vi "Logging Message Loop.vi"(8 "error in (no error)":errorcluster, 11 "Message Queues":T1) -> (0 "error out":errorcluster)   [LabVIEW 2021, in "Logging.lvlib"]
uses:
  Logging.lvlib
  Logging Configuration.ctl
  Logging State Cluster.ctl
  <vilib>/ErrorRing/Error Ring.xnode
  <vilib>/Utility/error.llb/Error Cluster From Error Code.vi
  Log State Enum.ctl
  Feed Module/Controls/Feed Module Shared Variable Cluster.ctl
  Feed Module/Feed Module.lvlib
  Settings Cluster.ctl
  Log Data Cluster.ctl
  support/Message Queue/Message Cluster.ctl
  support/Message Queue/All Message Queues.ctl
  support/Message Queue/Message Queue.lvlib
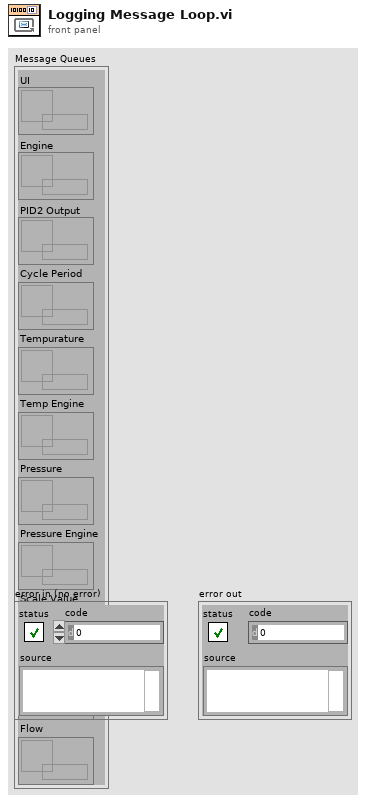
[diagram p1: front panel]
types:
  T1 = typedef "Message Queue.lvlib/All Message Queues.ctl" = cluster{"UI":refnum<queue>, "Engine":refnum<queue>, "PID2 Output":refnum<queue>, "Cycle Period":refnum<queue>, "Tempurature":refnum<queue>, "Temp Engine":refnum<queue>, "Pressure":refnum<queue>, "Pressure Engine":refnum<queue>, "Scale Value":refnum<queue>, "Pump Status":refnum<queue>, "Flow":refnum<queue>}
  T2 = typedef "Logging.lvlib/Logging State Cluster.ctl" = cluster{"State":T3, "File refnum":refnum<file>, "Start Time":timestamp, "Settings":T4, "Process Name":string, "First Record":bool}
  T3 = typedef "Logging.lvlib/Log State Enum.ctl" = enum16{"Logging", "Idle"}
  T4 = typedef "Logging.lvlib/Settings Cluster.ctl" = cluster{"Logging Configuration":T5, "Shared Variables":T6}
  T5 = typedef "Logging.lvlib/Logging Configuration.ctl" = cluster{"Log File Base Path":path}
  T6 = typedef "Feed Module.lvlib/Feed Module Shared Variable Cluster.ctl" = cluster{"PID 1 Process Variable":string, "PID 1 Output":string, "PID 1 Setpoint":string, "PID 1 Setpoint SV refnum":refnum<k21>, "PID 1 Process Variable SV refnum":refnum<k21>, "PID 1 Output SV refnum":refnum<k21>}
  T7 = enum16{"open", "replace", "create", "open or create", "replace or create", "replace or create with confirmation"}
  T8 = typedef "Logging.lvlib/Log Data Cluster.ctl" = cluster{"Time Stamp":timestamp, "PID 2 Output":dbl, "PID 2 Process Variable":dbl, "PID 1 Output":dbl}
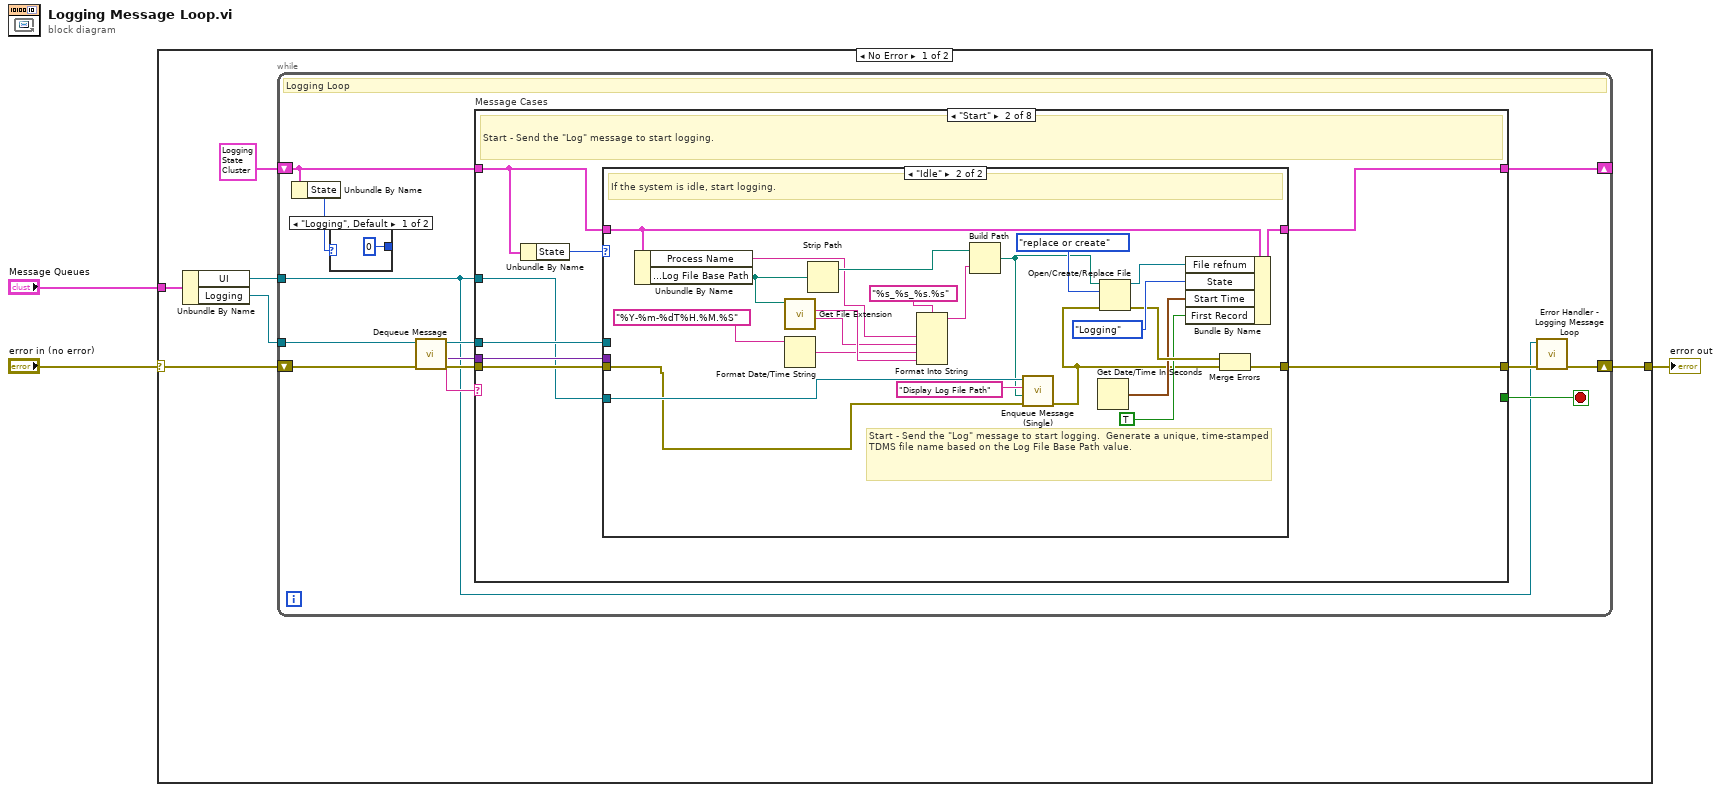
[diagram p0: block diagram]
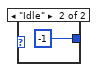
[diagram p2: hidden frame]
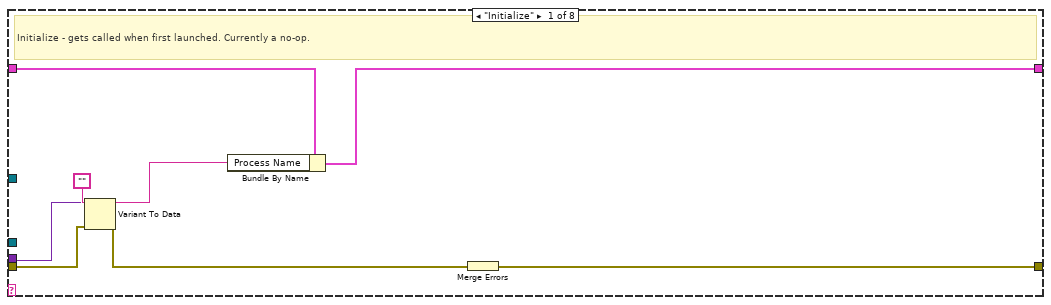
[diagram p3: hidden frame]
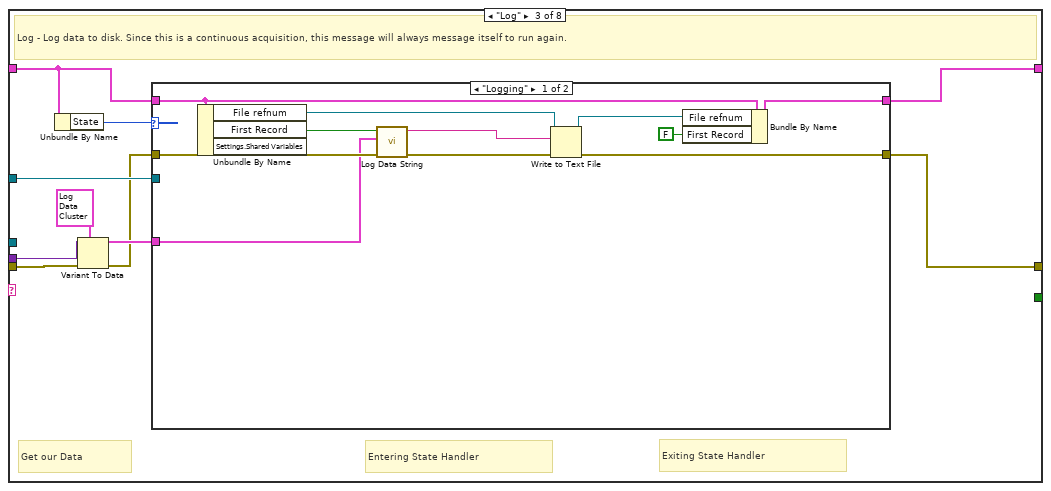
[diagram p5: hidden frame]
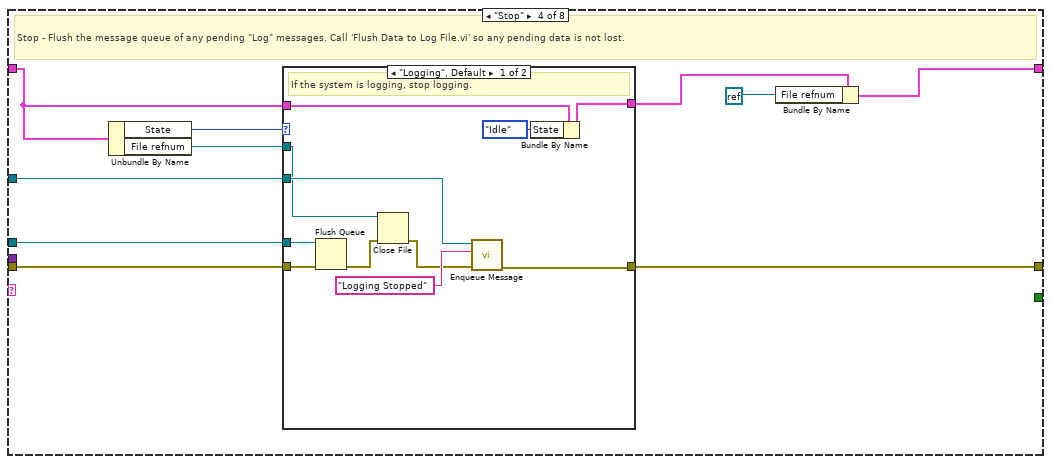
[diagram p7: hidden frame]
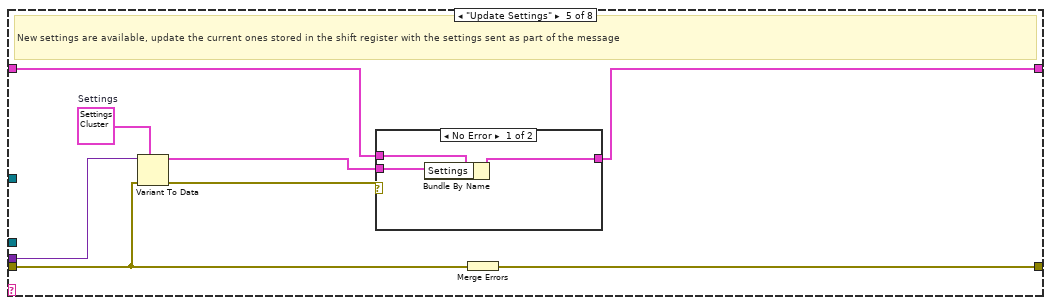
[diagram p9: hidden frame]
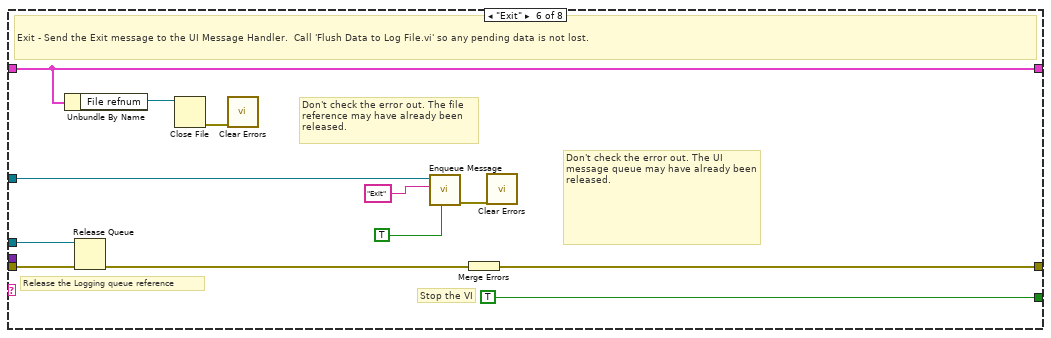
[diagram p11: hidden frame]
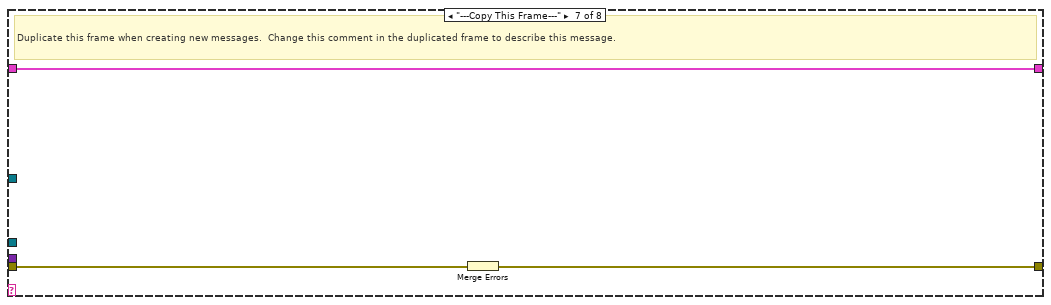
[diagram p12: hidden frame]
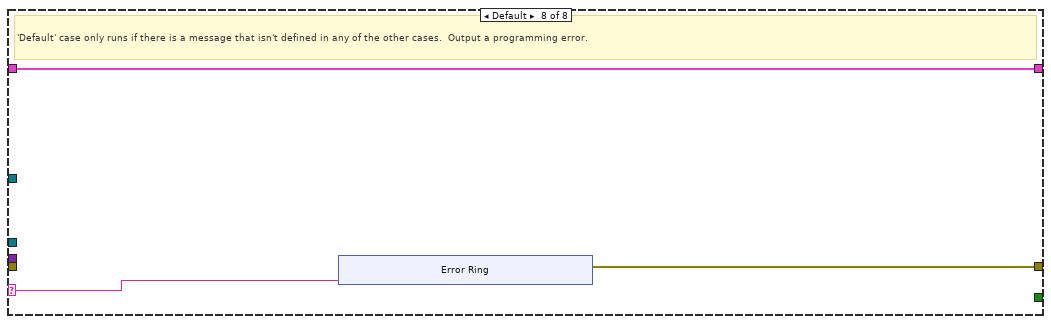
[diagram p13: hidden frame]
diagram:
  n1 = case shown="No Error" "error in (no error)" {
    selector: "error in (no error)" -> [w6 w149]
    tunnel: "Message Queues" -> [w9 _]
    tunnel: [w7 w149] -> w2
    frame No Error {
      n2 = Unbundle By Name(w9) -> ("UI"=w5:refnum<queue>, "Logging"=w8:refnum<queue>)
      n3 = while {
        tunnel: w8 -> [w16]
        shift-right: [w10] -> _
        shift-left: T2 {"State"=enum."Idle", "File refnum"=refnum, "Start Time"=timestamp(0 s since 1904-01-01), "Settings"={"Logging Configuration"={"Log File Base Path"=path ""}, "Shared Variables"={"PID 1 Process Variable"="PID1-Mettler Toledo Scale 1", "PID 1 Output"="PID1-Mettler Toledo Scale 1", "PID 1 Setpoint"="PID1-Setpoint", "PID 1 Setpoint SV refnum"="", "PID 1 Process Variable SV refnum"="", "PID 1 Output SV refnum"=""}}, "Process Name"="", "First Record"=FALSE} -> [w12]
        shift-right: [w14] -> w7
        shift-left: w6 -> [w21]
        tunnel: w5 -> [w13]
        stop <- w22 stop-if-true
        # "Logging Loop"
        n4 = Unbundle By Name(w12) -> ("State"=w11:T3)
        n5 = case shown="\"Logging\", Default" w11 {
          tunnel: [0 ("timeout in ms (-1)") -1 ("timeout in ms (-1)")] -> _
          frame "Logging", Default {
          }
          frame "Idle" {
          }
        }
        n6 = call "Dequeue Message.vi"("error in (no error)"=w21, "Message Queue"=w16) -> ("error out"=w20:errorcluster, "Message Data"=w18:variant, "Message"=w19:string, "dup Message Queue"=w17:refnum<queue>)  [unwired: 6 in]
        n7 = case "Message Cases" shown="\"Start\"" w19 {
          selector: w19 -> [_ _ _ _ _ _ _ w139]
          tunnel: w17 -> [_ w39 _ w96 _ w129 _ _]
          tunnel: w20 -> [w26 w38 w66 w97 w117 w132 w138 _]
          tunnel: [w32 w40 w73 w98 w119 w134 w136 w140] -> w15
          tunnel: w12 -> [w30 w34 w71 w91 w115 w127 w137 w141]
          tunnel: [w31 w37 w72 w95 w113 w127 w137 w141] -> w10
          tunnel: [_ _ _ _ _ TRUE _ _] -> w22
          tunnel: w18 -> [w28 w35 w70 _ w118 _ _ _]
          tunnel: w13 -> [_ w33 w74 w94 _ w133 _ _]
          frame "Initialize" {
            # "Initialize - gets called when first launched. Currently a no-op."
            n8 = Variant To Data(error in=w26, type="", Variant=w28) -> (data=w25:string, error out=w27:errorcluster)
            n9 = Bundle By Name(cluster=w30, "Process Name"=w25) -> (w31:T2)
            n10 = Merge Errors(w27) -> (w32:errorcluster)
          }
          frame "Start" {
            # "Start - Send the \"Log\" message to start logging."
            n11 = Unbundle By Name(w34) -> ("State"=w36:T3)
            n12 = case shown="\"Idle\"" w36 {
              tunnel: [w41 w65] -> w40
              tunnel: w39 -> [_ _]
              tunnel: w38 -> [w41 w43]
              tunnel: w34 -> [w42 w60]
              tunnel: [w42 w59] -> w37
              tunnel: w35 -> [_ _]
              tunnel: w33 -> [_ w47]
              frame "Logging", Default {
                # "The system is already running. Ignore the \"Start\" message."
              }
              frame "Idle" {
                # "Start - Send the \"Log\" message to start logging.  Generate a unique, time-stamped TDMS file name based on the Log File Base Path value."
                # "If the system is idle, start logging."
                n13 = Unbundle By Name(w60) -> ("Process Name"=w49:string, "Settings.Logging Configuration.Log File Base Path"=w54:path)
                n14 = call <vilib>:"Get File Extension.vi"("file"=w54) -> ("filename without extension"=w50:string, "lowercase file extension"=w62:string)  [unwired: 6 in, 3 out]
                n15 = Format Date/Time String(time format string (%c)="%Y-%m-%dT%H.%M.%S") -> (date/time string=w51:string)  [unwired: 2 in]
                n16 = Strip Path(path=w54) -> (stripped path=w53:path)  [unwired: 1 out]
                n17 = Format Into String(format string="%s_%s_%s.%s", w49, w50, w51, w62) -> (resulting string=w61:string)  [unwired: 2 in, 1 out]
                n18 = Build Path(base path=w53, name or relative path=w61) -> (appended path=w45:path)
                n19 = call "Enqueue Message (Single).vi"("error in (no error)"=w43, "Message Data"=w45, "Message"="Display Log File Path", "Message Queue"=w47) -> ("error out"=w44:errorcluster)  [unwired: 6 in, 1 out]
                n20 = Get Date/Time In Seconds() -> (seconds since 1Jan1904=w52:timestamp)
                n21 = Open/Create/Replace File(file path (use dialog)=w45, error in=w44, operation (0:open)=T7."replace or create") -> (refnum out=w56:refnum<file>, error out=w57:errorcluster)  [unwired: 3 in, 1 out]
                n22 = Bundle By Name(cluster=w60, "File refnum"=w56, "State"=Log_State_Enum."Logging", "Start Time"=w52, "First Record"=TRUE) -> (w59:T2)
                n23 = Merge Errors(w57, w44) -> (w65:errorcluster)
              }
            }
          }
          frame "Log" {
            # "Exiting State Handler"
            # "Entering State Handler"
            # "Get our Data"
            # "Log - Log data to disk. Since this is a continuous acquisition, this message will always message itself to run again."
            n24 = Unbundle By Name(w71) -> ("State"=w75:T3)
            n25 = Variant To Data(error in=w66, type=T8 {"Time Stamp"=timestamp(0 s since 1904-01-01), "PID 2 Output"=0.0, "PID 2 Process Variable"=0.0, "PID 1 Output"=0.0} ("Log Data Cluster"), Variant=w70) -> (data=w68:T8, error out=w67:errorcluster)
            n26 = case shown="\"Logging\"" w75 {
              tunnel: w67 -> [w80 w88]
              tunnel: w71 -> [w84 w87]
              tunnel: w74 -> [_ _]
              tunnel: [w86 w88] -> w73
              tunnel: [w82 w87] -> w72
              tunnel: w68 -> [w78 _]
              frame "Logging" {
                n27 = Unbundle By Name(w84) -> ("File refnum"=w85:refnum<file>, "First Record"=w76:bool)  [unwired: 1 out]
                n28 = call "Log Data String.vi"("error in (no error)"=w80, "Log Data Cluster"=w78, "First Record"=w76) -> ("error out"=w81:errorcluster, "Log Data String"=w79:string)  [unwired: 7 in]
                n29 = Write to Text File(file (use dialog)=w85, text=w79, error in=w81) -> (refnum out=w83:refnum<file>, error out=w86:errorcluster)  [unwired: 1 in, 1 out]
                n30 = Bundle By Name(cluster=w84, "File refnum"=w83, "First Record"=FALSE) -> (w82:T2)
              }
              frame "Idle", Default {
              }
            }
          }
          frame "Stop" {
            # "Stop - Flush the message queue of any pending \"Log\" messages. Call 'Flush Data to Log File.vi' so any pending data is not lost."
            n31 = Unbundle By Name(w91) -> ("State"=w93:T3, "File refnum"=w90:refnum<file>)
            n32 = case shown="\"Logging\", Default" w93 {
              tunnel: [w102 w111] -> w98
              tunnel: w97 -> [w109 w111]
              tunnel: w96 -> [w108 _]
              tunnel: w94 -> [w107 _]
              tunnel: w91 -> [w105 w110]
              tunnel: [w104 w110] -> w92
              tunnel: w90 -> [w101 _]
              frame "Logging", Default {
                # "If the system is logging, stop logging."
                n33 = Flush Queue(queue=w108, error in (no error)=w109) -> (error out=w100:errorcluster)  [unwired: 2 out]
                n34 = Close File(refnum=w101, error in=w100) -> (error out=w99:errorcluster)  [unwired: 1 out]
                n35 = call-poly "Enqueue Message.vi"("error in (no error)"=w99, "Message"="Logging Stopped", "Message Queue"=w107) -> ("error out"=w102:errorcluster)  [unwired: 7 in, 1 out]
                n36 = Bundle By Name(cluster=w105, "State"=Log_State_Enum."Idle") -> (w104:T2)
              }
              frame "Idle" {
                # "The system is already idle. Ignore the \"Stop\" message."
              }
            }
            n37 = Bundle By Name(cluster=w92, "File refnum"=refnum<k0> refnum) -> (w95:T2)
          }
          frame "Update Settings" {
            w112 = T4 {"Logging Configuration"={"Log File Base Path"=path ""}, "Shared Variables"={"PID 1 Process Variable"="PID1-Mettler Toledo Scale 1", "PID 1 Output"="PID1-Mettler Toledo Scale 1", "PID 1 Setpoint"="PID1-Setpoint", "PID 1 Setpoint SV refnum"="", "PID 1 Process Variable SV refnum"="", "PID 1 Output SV refnum"=""}}  # Settings
            # "New settings are available, update the current ones stored in the shift register with the settings sent as part of the message"
            n38 = Variant To Data(error in=w117, type=w112, Variant=w118) -> (data=w114:T4, error out=w116:errorcluster)
            n39 = case shown="No Error" w116 {
              tunnel: w115 -> [w122 w123]
              tunnel: w114 -> [w121 _]
              tunnel: [w120 w123] -> w113
              frame No Error {
                n40 = Bundle By Name(cluster=w122, "Settings"=w121) -> (w120:T2)
              }
              frame Error {
              }
            }
            n41 = Merge Errors(w117) -> (w119:errorcluster)
          }
          frame "Exit" {
            # "Don't check the error out. The file reference may have already been released."
            # "Release the Logging queue reference"
            # "Don't check the error out. The UI message queue may have already been released."
            # "Stop the VI"
            # "Exit - Send the Exit message to the UI Message Handler.  Call 'Flush Data to Log File.vi' so any pending data is not lost."
            n42 = Unbundle By Name(w127) -> ("File refnum"=w126:refnum<file>)
            n43 = Release Queue(queue=w129, error in (no error)=w132) -> (error out=w128:errorcluster)  [unwired: 1 in, 2 out]
            n44 = Close File(refnum=w126) -> (error out=w125:errorcluster)  [unwired: 1 in, 1 out]
            n45 = call <vilib>:"Clear Errors.vi"("error in (no error)"=w125) -> ()  [unwired: 5 in, 2 out]
            n46 = call-poly "Enqueue Message.vi"("Priority Message? (F)"=TRUE, "Message"="Exit", "Message Queue"=w133) -> ("error out"=w124:errorcluster)  [unwired: 7 in, 1 out]
            n47 = Merge Errors(w128) -> (w134:errorcluster)
            n48 = call <vilib>:"Clear Errors.vi"("error in (no error)"=w124) -> ()  [unwired: 5 in, 2 out]
          }
          frame "---Copy This Frame---" {
            # "Duplicate this frame when creating new messages.  Change this comment in the duplicated frame to describe this message."
            n49 = Merge Errors(w138) -> (w136:errorcluster)
          }
          frame Default {
            # "'Default' case only runs if there is a message that isn't defined in any of the other cases.  Output a programming error."
            n50 = xnode "Error Ring"("parameter 0"=w139) -> ("error out"=w140:errorcluster)
          }
        }
        n51 = call "Error Handler - Logging Message Loop.vi"("error in (no error)"=w15, "Message Queue"=w13) -> ("dup error in"=w14:errorcluster)  [unwired: 8 in, 1 out]
      }
    }
    frame Error {
    }
  }
  "error out" <- w2
